vi "id.To JSON String.vi"(8 "error in (no error)":errorcluster, 11 "id in":refnum<class "id.lvclass">) -> (0 "error out":errorcluster, 2 "JSON String":string, 3 "id out":refnum<class "id.lvclass">)   [LabVIEW 2020, in "JSON-RPC Lib.lvlib" / "id.lvclass"]
uses:
  id.lvclass
  Variant JSON API/Variant JSON API.lvlib
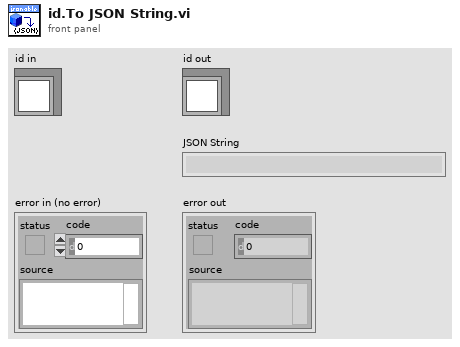
[diagram p1: front panel]
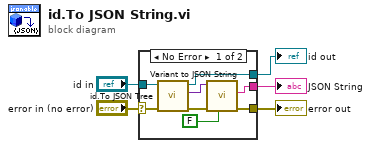
[diagram p0: block diagram]
diagram:
  n1 = case shown="No Error" "error in (no error)" {
    selector: "error in (no error)" -> [w12 w15]
    tunnel: [w9 w15] -> w4
    tunnel: [w11 w14] -> w2
    tunnel: "id in" -> [w13 w14]
    tunnel: [w10 _] -> w1
    frame No Error {
      n2 = call "id.To JSON Tree.vi"("error in (no error)"=w12, "id in"=w13) -> ("error out"=w8:errorcluster, "JSON Value out"=w6:variant, "id out"=w11:refnum<class "id.lvclass">)  [unwired: 7 in]
      n3 = call "Variant to JSON String.vi"("pretty print? (F)"=FALSE ("pretty print? (T)"), "error in (no error)"=w8, "Variant in"=w6) -> ("error out"=w9:errorcluster, "String"=w10:string)  [unwired: 6 in, 1 out]
    }
    frame Error {
    }
  }
  "error out" <- w4
  "id out" <- w2
  "JSON String" <- w1
